vi "应用事件编程.vi"() -> ()   [LabVIEW 2010]
panel:
  in  "确定按钮":bool
  # "按F2后击键"
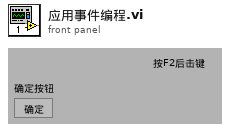
[diagram p1: front panel]
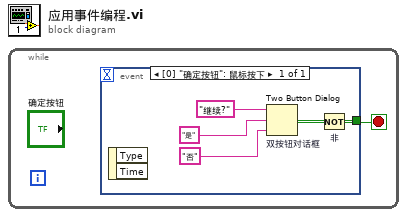
[diagram p0: block diagram]
diagram:
  n1 = while {
    stop <- w1 stop-if-true
    n2 = event shown="[0] \"确定按钮\": 鼠标按下" {
      selector: _ -> [_]
      dyn-events: _ -> [_]
      timeout: _ -> [_]
      tunnel: [w2] -> w1
      event "确定按钮": Mouse Down {
        n3 = event-data() -> ()  [unwired: 1 in, 2 out]
        n4 = Two Button Dialog "双按钮对话框"(message="继续?", 1:"否" ("F button name (\"Cancel\")"), 2:"是" ("T button name (\"OK\")")) -> (T button?=w5:bool)
        n5 = Not "非"(x=w5) -> (.not. x?=w2:bool)
      }
    }
  }
